vi "Com_SECS Equipment _Message Data Encoding.vi"(8 "error in":errorcluster, 11 "Message Data In":T1[](array[typedef])) -> (0 "error out":errorcluster, 3 "Message Data Out":u8[](array[numeric]))   [LabVIEW 2016]
uses:
  Data Def/Com_SECS Equipment _Message Data.ctl
  Data Def/Com_SECS Equipment _Data Item Format.ctl
  Data Def/Com_SECS Equipment _Format Code.ctl
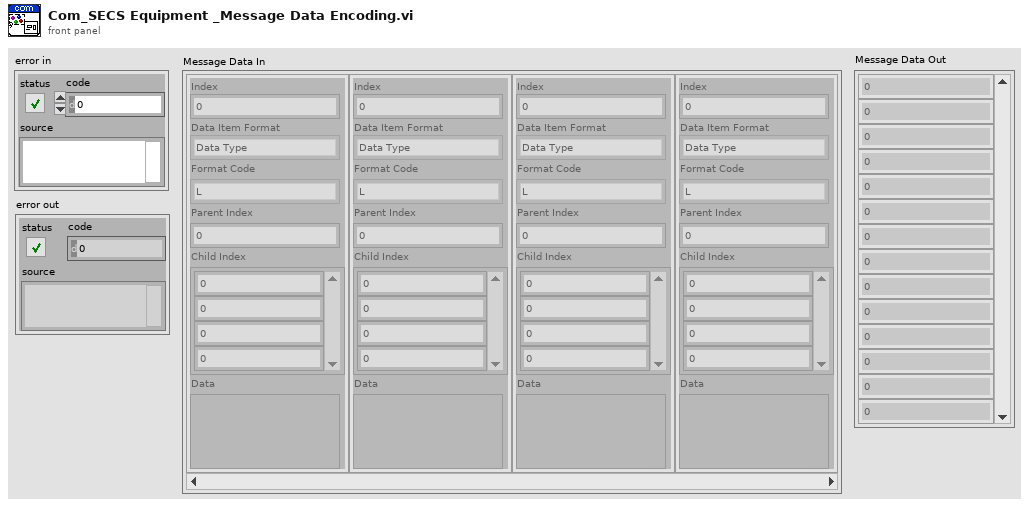
[diagram p1: front panel]
types:
  T1 = typedef "Com_SECS Equipment _Message Data.ctl" = cluster{"Index":i32, "Data Item Format":T2, "Format Code":T3, "Parent Index":i32, "Child Index":i32[], "Data":variant}
  T2 = typedef "Com_SECS Equipment _Data Item Format.ctl" = enum16{"Data Type", "Value"}
  T3 = typedef "Com_SECS Equipment _Format Code.ctl" = enum16{"L", "A", "B", "Boolean", "J", "I1", "I2", "I4", "I8", "U1", "U2", "U4", "U8", "F4", "F8", "Char"}
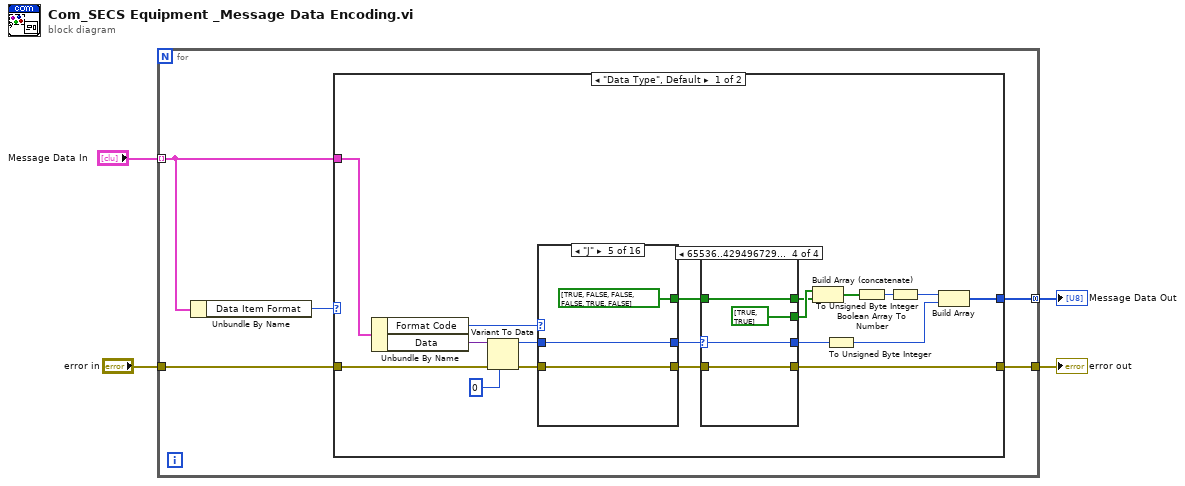
[diagram p0: block diagram]
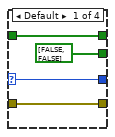
[diagram p2: hidden frame]
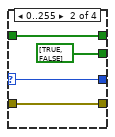
[diagram p3: hidden frame]
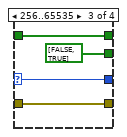
[diagram p4: hidden frame]
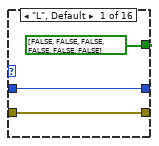
[diagram p5: hidden frame]
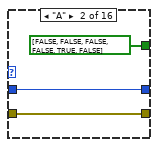
[diagram p6: hidden frame]
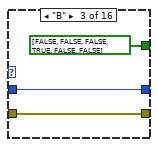
[diagram p7: hidden frame]
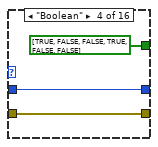
[diagram p8: hidden frame]
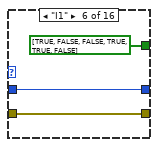
[diagram p9: hidden frame]
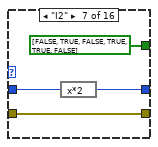
[diagram p10: hidden frame]
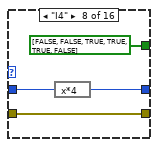
[diagram p11: hidden frame]
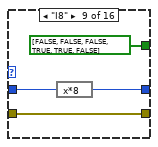
[diagram p12: hidden frame]
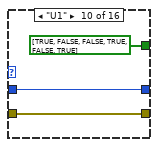
[diagram p13: hidden frame]
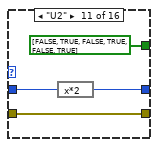
[diagram p14: hidden frame]
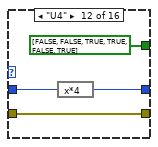
[diagram p15: hidden frame]
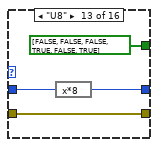
[diagram p16: hidden frame]
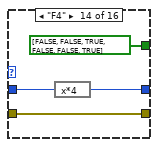
[diagram p17: hidden frame]
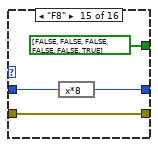
[diagram p18: hidden frame]
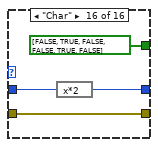
[diagram p19: hidden frame]
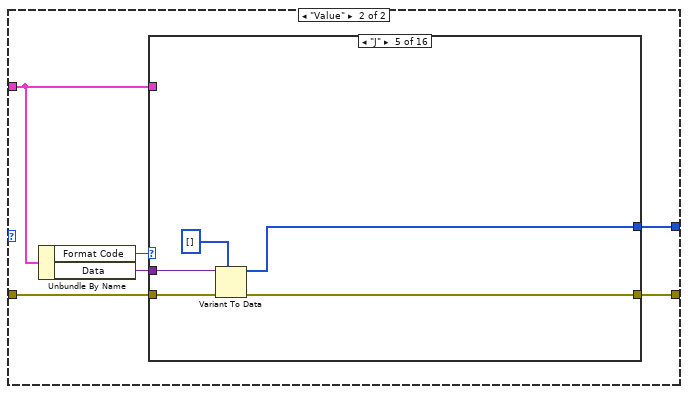
[diagram p20: hidden frame]
diagram:
  n1 = for {
    tunnel: "Message Data In" -> [w7] mode=indexing
    tunnel: "error in" -> [w8]
    tunnel: [w6] -> w1 mode=concatenating
    tunnel: [w5] -> w2
    n2 = Unbundle By Name(w7) -> ("Data Item Format"=w9:T2)
    n3 = case shown="\"Data Type\", Default" w9 {
      tunnel: w8 -> [w27 w106]
      tunnel: w7 -> [w12 w105]
      tunnel: [w14 w102] -> w6
      tunnel: [w13 w103] -> w5
      frame "Data Type", Default {
        n4 = Unbundle By Name(w12) -> ("Format Code"=w24:T3, "Data"=w26:variant)
        n5 = Variant To Data(error in=w27, type=u32 0 ("Data Length"), Variant=w26) -> (data=w23:u32, error out=w25:errorcluster)
        n6 = case shown="\"J\"" w24 {
          tunnel: w25 -> [w45 w49 w52 w55 w58 w61 w66 w70 w74 w76 w81 w85 w89 w93 w97 w101]
          tunnel: w23 -> [w46 w50 w53 w56 w59 w62 w64 w68 w72 w77 w79 w83 w87 w91 w95 w99]
          tunnel: [bool[] [FALSE, FALSE, FALSE, FALSE, FALSE, FALSE] bool[] [FALSE, FALSE, FALSE, FALSE, TRUE, FALSE] bool[] [FALSE, FALSE, FALSE, TRUE, FALSE, FALSE] bool[] [TRUE, FALSE, FALSE, TRUE, FALSE, FALSE] bool[] [TRUE, FALSE, FALSE, FALSE, TRUE, FALSE] bool[] [TRUE, FALSE, FALSE, TRUE, TRUE, FALSE] bool[] [FALSE, TRUE, FALSE, TRUE, TRUE, FALSE] bool[] [FALSE, FALSE, TRUE, TRUE, TRUE, FALSE] bool[] [FALSE, FALSE, FALSE, TRUE, TRUE, FALSE] bool[] [TRUE, FALSE, FALSE, TRUE, FALSE, TRUE] bool[] [FALSE, TRUE, FALSE, TRUE, FALSE, TRUE] bool[] [FALSE, FALSE, TRUE, TRUE, FALSE, TRUE] bool[] [FALSE, FALSE, FALSE, TRUE, FALSE, TRUE] bool[] [FALSE, FALSE, TRUE, FALSE, FALSE, TRUE] bool[] [FALSE, FALSE, FALSE, FALSE, FALSE, TRUE] bool[] [FALSE, TRUE, FALSE, FALSE, TRUE, FALSE]] -> w20
          tunnel: [w46 w50 w53 w56 w59 w62 w63 w67 w71 w77 w78 w82 w86 w90 w94 w98] -> w21
          tunnel: [w45 w49 w52 w55 w58 w61 w66 w70 w74 w76 w81 w85 w89 w93 w97 w101] -> w22
          frame "L", Default {
          }
          frame "A" {
          }
          frame "B" {
          }
          frame "Boolean" {
          }
          frame "J" {
          }
          frame "I1" {
          }
          frame "I2" {
            n7 = expression code="x*2"(w64) -> (w63:u32)
          }
          frame "I4" {
            n8 = expression code="x*4"(w68) -> (w67:u32)
          }
          frame "I8" {
            n9 = expression code="x*8"(w72) -> (w71:u32)
          }
          frame "U1" {
          }
          frame "U2" {
            n10 = expression code="x*2"(w79) -> (w78:u32)
          }
          frame "U4" {
            n11 = expression code="x*4"(w83) -> (w82:u32)
          }
          frame "U8" {
            n12 = expression code="x*8"(w87) -> (w86:u32)
          }
          frame "F4" {
            n13 = expression code="x*4"(w91) -> (w90:u32)
          }
          frame "F8" {
            n14 = expression code="x*8"(w95) -> (w94:u32)
          }
          frame "Char" {
            n15 = expression code="x*2"(w99) -> (w98:u32)
          }
        }
        n16 = case shown="65536..4294967295" w21 {
          selector: w21 -> [w29 w33 w37 w41]
          tunnel: w22 -> [w32 w36 w40 w44]
          tunnel: [w32 w36 w40 w44] -> w13
          tunnel: [bool[] [FALSE, FALSE] bool[] [TRUE, FALSE] bool[] [FALSE, TRUE] bool[] [TRUE, TRUE]] -> w19
          tunnel: w20 -> [w30 w34 w38 w42]
          tunnel: [w30 w34 w38 w42] -> w18
          tunnel: [w29 w33 w37 w41] -> w11
          frame Default {
          }
          frame 0..255 {
          }
          frame 256..65535 {
          }
          frame 65536..-1 {
          }
        }
        n17 = Build Array (concatenate)(w19, w18) -> (w17:bool[])
        n18 = To Unsigned Byte Integer(number=w11) -> (unsigned 8bit integer=w10:u8)
        n19 = Boolean Array To Number(Boolean array=w17) -> (number=w16:u32)
        n20 = To Unsigned Byte Integer(number=w16) -> (unsigned 8bit integer=w15:u8)
        n21 = Build Array(w15, w10) -> (w14:u8[])
      }
      frame "Value" {
        n22 = Unbundle By Name(w105) -> ("Format Code"=w107:T3, "Data"=w104:variant)
        n23 = case shown="\"J\"" w107 {
          tunnel: w106 -> [w108 w114 w120 w131 w136 w142 w149 w159 w169 w177 w184 w194 w204 w214 w224 w233]
          tunnel: w105 -> [_ _ _ _ _ _ _ _ _ _ _ _ _ _ _ _]
          tunnel: w104 -> [_ w113 w119 w130 w135 w141 w148 w158 w168 w176 w183 w193 w203 w213 w223 w232]
          tunnel: [w108 w111 w118 w129 w134 w140 w147 w157 w167 w175 w182 w192 w202 w212 w222 w231] -> w103
          tunnel: [_ w109 w115 w125 w132 w137 w143 w153 w163 w173 w178 w188 w198 w208 w218 w228] -> w102
          frame "L", Default {
          }
          frame "A" {
            n24 = Variant To Data(error in=w114, type="", Variant=w113) -> (data=w110:string, error out=w111:errorcluster)
            n25 = String To Byte Array(string=w110) -> (unsigned byte array=w109:u8[])
          }
          frame "B" {
            n26 = Variant To Data(error in=w120, type=cluster{bool[]}[] [], Variant=w119) -> (data=w116:cluster{bool[]}[], error out=w118:errorcluster)
            n27 = for {
              tunnel: w116 -> [w124] mode=indexing
              tunnel: [w121] -> w115 mode=indexing
              n28 = Unbundle(w124) -> (w123:bool[])
              n29 = Boolean Array To Number(Boolean array=w123) -> (number=w122:u32)
              n30 = To Unsigned Byte Integer(number=w122) -> (unsigned 8bit integer=w121:u8)
            }
          }
          frame "Boolean" {
            n31 = Variant To Data(error in=w131, type=bool[] [], Variant=w130) -> (data=w127:bool[], error out=w129:errorcluster)
            n32 = Boolean To (0,1)(Boolean=w127) -> (0, 1=w126:i16[])
            n33 = To Unsigned Byte Integer(number=w126) -> (unsigned 8bit integer=w125:u8[])
          }
          frame "J" {
            n34 = Variant To Data(error in=w136, type=u8[] [], Variant=w135) -> (data=w132:u8[], error out=w134:errorcluster)
          }
          frame "I1" {
            n35 = Variant To Data(error in=w142, type=i8[] [], Variant=w141) -> (data=w138:i8[], error out=w140:errorcluster)
            n36 = To Unsigned Byte Integer(number=w138) -> (unsigned 8bit integer=w137:u8[])
          }
          frame "I2" {
            n37 = Variant To Data(error in=w149, type=i16[] [], Variant=w148) -> (data=w145:i16[], error out=w147:errorcluster)
            n38 = for {
              tunnel: w145 -> [w152] mode=indexing
              tunnel: u8[] [] -> [w151]
              tunnel: [w150] -> w143 mode=concatenating
              n39 = Type Cast(type=w151, x=w152) -> (*(type *) &x=w150:u8[])
            }
          }
          frame "I4" {
            n40 = Variant To Data(error in=w159, type=i32[] [], Variant=w158) -> (data=w155:i32[], error out=w157:errorcluster)
            n41 = for {
              tunnel: w155 -> [w162] mode=indexing
              tunnel: u8[] [] -> [w161]
              tunnel: [w160] -> w153 mode=concatenating
              n42 = Type Cast(type=w161, x=w162) -> (*(type *) &x=w160:u8[])
            }
          }
          frame "I8" {
            n43 = Variant To Data(error in=w169, type=i64[] [], Variant=w168) -> (data=w165:i64[], error out=w167:errorcluster)
            n44 = for {
              tunnel: w165 -> [w172] mode=indexing
              tunnel: u8[] [] -> [w171]
              tunnel: [w170] -> w163 mode=concatenating
              n45 = Type Cast(type=w171, x=w172) -> (*(type *) &x=w170:u8[])
            }
          }
          frame "U1" {
            n46 = Variant To Data(error in=w177, type=u8[] [], Variant=w176) -> (data=w173:u8[], error out=w175:errorcluster)
          }
          frame "U2" {
            n47 = Variant To Data(error in=w184, type=u16[] [], Variant=w183) -> (data=w180:u16[], error out=w182:errorcluster)
            n48 = for {
              tunnel: w180 -> [w187] mode=indexing
              tunnel: u8[] [] -> [w186]
              tunnel: [w185] -> w178 mode=concatenating
              n49 = Type Cast(type=w186, x=w187) -> (*(type *) &x=w185:u8[])
            }
          }
          frame "U4" {
            n50 = Variant To Data(error in=w194, type=u32[] [], Variant=w193) -> (data=w190:u32[], error out=w192:errorcluster)
            n51 = for {
              tunnel: w190 -> [w197] mode=indexing
              tunnel: u8[] [] -> [w196]
              tunnel: [w195] -> w188 mode=concatenating
              n52 = Type Cast(type=w196, x=w197) -> (*(type *) &x=w195:u8[])
            }
          }
          frame "U8" {
            n53 = Variant To Data(error in=w204, type=u64[] [], Variant=w203) -> (data=w200:u64[], error out=w202:errorcluster)
            n54 = for {
              tunnel: w200 -> [w207] mode=indexing
              tunnel: u8[] [] -> [w206]
              tunnel: [w205] -> w198 mode=concatenating
              n55 = Type Cast(type=w206, x=w207) -> (*(type *) &x=w205:u8[])
            }
          }
          frame "F4" {
            n56 = Variant To Data(error in=w214, type=sgl[] [], Variant=w213) -> (data=w210:sgl[], error out=w212:errorcluster)
            n57 = for {
              tunnel: w210 -> [w217] mode=indexing
              tunnel: u8[] [] -> [w216]
              tunnel: [w215] -> w208 mode=concatenating
              n58 = Type Cast(type=w216, x=w217) -> (*(type *) &x=w215:u8[])
            }
          }
          frame "F8" {
            n59 = Variant To Data(error in=w224, type=dbl[] [], Variant=w223) -> (data=w220:dbl[], error out=w222:errorcluster)
            n60 = for {
              tunnel: w220 -> [w227] mode=indexing
              tunnel: u8[] [] -> [w226]
              tunnel: [w225] -> w218 mode=concatenating
              n61 = Type Cast(type=w226, x=w227) -> (*(type *) &x=w225:u8[])
            }
          }
          frame "Char" {
            n62 = Variant To Data(error in=w233, type="", Variant=w232) -> (data=w229:string, error out=w231:errorcluster)
            n63 = String To Byte Array(string=w229) -> (unsigned byte array=w228:u8[])
          }
        }
      }
    }
  }
  "error out" <- w2
  "Message Data Out" <- w1
